vi "Init.vi"(8 "error in (no error)":errorcluster, 10 "Address":string, 11 "HRS_Spectrometer in":refnum<class "HRS_Spectrometer.lvclass">) -> (0 "error out":errorcluster, 3 "HRS_Spectrometer out":refnum<class "HRS_Spectrometer.lvclass">)   [LabVIEW 2023, in "HRS_Spectrometer.lvlib" / "HRS_Spectrometer.lvclass"]
uses:
  HRS_Spectrometer.lvclass
  Applications/National Instruments/LabVIEW 2023 64-bit/vi.lib/ActorFramework/Actor/Actor.lvclass
  <vilib>/ActorFramework/Actor/Actor.lvclass/Actor.ctl
  <vilib>/Instr/_visa.llb/Select Event Type.ctl
  HRS_Spectrometer.lvclass/HRS_Spectrometer.ctl
  Interfaces/InitDeinitInterface/InitDeinitComm Messages/InitDone Msg/InitDone Msg.lvclass/InitDone Msg.ctl
  <vilib>/ActorFramework/Message Enqueuer/Message Enqueuer.lvclass/Message Enqueuer.ctl
  <vilib>/ActorFramework/Message Enqueuer/Enqueue.vi
  Interfaces/InitDeinitInterface/InitDeinitComm Messages/InitDone Msg/InitDone Msg.lvclass
  Applications/National Instruments/LabVIEW 2023 64-bit/vi.lib/ActorFramework/Message/Message.lvclass
  <vilib>/ActorFramework/Message Priority Queue/Priority Enqueue.vi
  <vilib>/ActorFramework/Actor/Actor.lvclass
  Users/alexandrosspiliotis/Documents/LV_DAQ_Project/ConcreteClasses/ConcreteInstrumentClasses/SpectrometerClasses/Spectrometer_HRS_LV/HRS_Spectrometer/HRS_Spectrometer/HRS_Spectrometer.lvclass
  Users/alexandrosspiliotis/Documents/LV_DAQ_Project/Interfaces/InitDeinitInterface/InitDeinit/InitDeinit.lvclass
  Users/alexandrosspiliotis/Documents/LV_DAQ_Project/Interfaces/AbstractInstrumentClasses/Spectrometers_LV/SpectrometerInterface/Spectrometer.lvclass
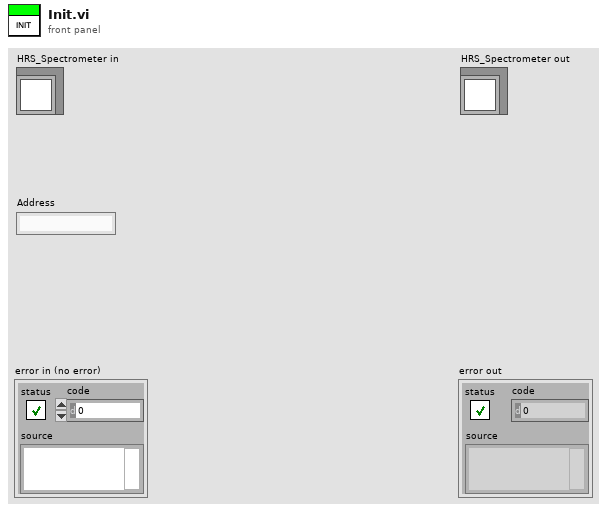
[diagram p1: front panel]
types:
  T1 = typedef "Select Event Type.ctl" = u32
  T2 = typedef "instrumentType.ctl" = enum16{"Spectrometer", "Camera", "Stepper"}
  T3 = cluster{"address type":enum16{"VISA", "Index"}, string, "instrument type":T2}
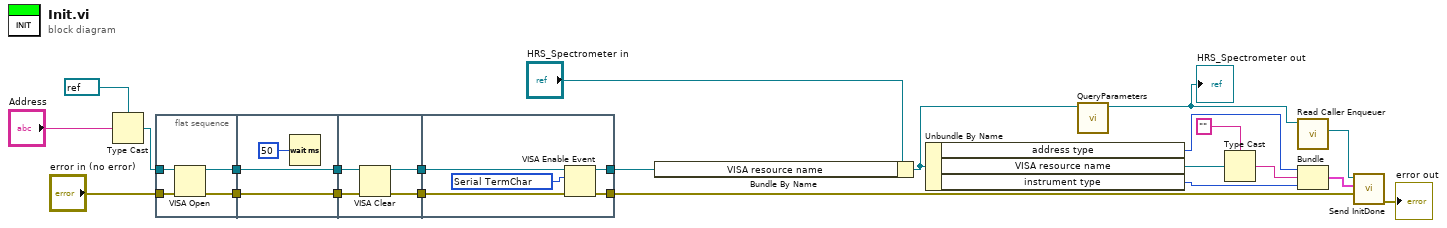
[diagram p0: block diagram]
diagram:
  n1 = Type Cast(type=refnum<visa-resource-name> refnum ("VISA resource name"), x="Address") -> (*(type *) &x=w22:refnum<visa-resource-name>)
  n2 = flat-sequence {
    tunnel: w22 -> [w27]
    tunnel: "error in (no error)" -> [w26]
    tunnel: [w25] -> w20
    tunnel: [w24] -> w18
    tunnel: w20 -> [w29]
    tunnel: [w29] -> w19
    tunnel: w18 -> [w28]
    tunnel: [w28] -> w17
    tunnel: w19 -> [w34]
    tunnel: w17 -> [w33]
    tunnel: [w32] -> w13
    tunnel: [w31] -> w12
    tunnel: [w37] -> w8
    tunnel: [w35] -> w15
    tunnel: w13 -> [w36]
    tunnel: w12 -> [w38]
    frame #0 {
      n3 = VISA Open(error in (no error)=w26, VISA resource name=w27) -> (VISA resource name=w25:refnum<visa-resource-name>, error out=w24:errorcluster)  [unwired: 3 in]
    }
    frame #1 {
      n4 = Wait (ms)(milliseconds to wait=u32 50) -> ()  [unwired: 1 out]
    }
    frame #2 {
      n5 = VISA Clear(VISA resource name=w34, error in (no error)=w33) -> (VISA resource name out=w31:refnum<visa-resource-name>, error out=w32:errorcluster)
    }
    frame #3 {
      w39 = T1 1073684516 items=["Service Request"=1073684491, "Trigger"=3221168138, "Clear"=1073684493, "VXI Signal"=1073684512, "VXI/VME Interrupt"=3221168161, "VXI/VME Sysfail"=1073684509, "VXI/VME Sysreset"=1073684510, "GPIB CIC"=1073684498, "GPIB Talk"=1073684499, "GPIB Listen"=1073684500, "PXI Interrupt"=1073684514, "Serial Break"=1073684515, "Serial TermChar"=1073684516, "Serial CTS"=1073684521, "Serial DSR"=1073684522, "Serial DCD"=1073684524, "Serial RI"=1073684526, "Serial Character"=1073684533, "USB Interrupt"=1073684535, "All Enabled"=1073709055] ("Event Type")
      n6 = VISA Enable Event(8:w36, 10:w39, 11:w38) -> (0:w35:errorcluster, 3:w37:refnum<visa-resource-name>)  [unwired: 1 in]
    }
  }
  n7 = Bundle By Name(cluster="HRS_Spectrometer in", "VISA resource name"=w8) -> (w7:refnum<class "HRS_Spectrometer.lvclass">)
  n8 = Unbundle By Name(w7) -> ("address type"=w5:enum16{"VISA", "Index"}, "VISA resource name"=w3:refnum<visa-resource-name>, "instrument type"=w6:T2)
  n9 = call-dynamic "QueryParameters.vi"("HRS_Spectrometer in"=w7) -> ("HRS_Spectrometer out"=w4:refnum<class "HRS_Spectrometer.lvclass">)  [unwired: 9 in, 1 out]
  "HRS_Spectrometer out" <- w4
  n10 = Type Cast(type="", x=w3) -> (*(type *) &x=w2:string)
  n11 = call <vilib>:"Read Caller Enqueuer.vi"("Actor"=w4) -> ("Caller Enqueuer"=w16:refnum<class "Message Enqueuer.lvclass">)  [unwired: 10 in]
  n12 = Bundle("address type"=w5, w2, "instrument type"=w6) -> (w10:T3)  [unwired: 1 in]
  n13 = call "Send InitDone.vi"("instr error"=w15, "Address"=w10, "Message Enqueuer"=w16) -> ("error out"=→"error out":errorcluster)  [unwired: 7 in, 1 out]
